vi "瀑布显示.vi"(1 "报文信息记录":string[][](array[string])) -> (15 "显示":string)   [LabVIEW 2019]
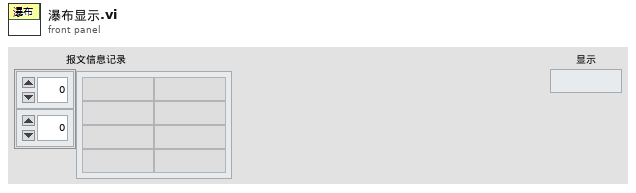
[diagram p1: front panel]
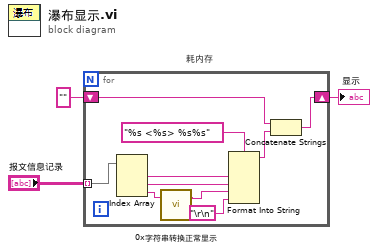
[diagram p0: block diagram]
diagram:
  # "耗内存"
  n1 = for {
    tunnel: "报文信息记录" -> [w13] mode=indexing
    shift-right: [w7] -> w1
    shift-left: "" -> [w6]
    n2 = Index Array(array=w13) -> (element #1=w12:string, element #2=w11:string, element #3=w4:string)  [unwired: 3 in]
    n3 = call "0x字符串转换正常显示.vi"("普通字符串"=w4) -> ("0x普通字符串"=w5:string)  [unwired: 18 in]
    n4 = Format Into String(format string="%s <%s> %s%s" ("格式字符串"), w12, w11, w5, "\r\n") -> (resulting string=w8:string)  [unwired: 2 in, 1 out]
    n5 = Concatenate Strings(w6, w8) -> (w7:string)
  }
  "显示" <- w1
